vi "Save text file.vi"(8 "error in (no error)":errorcluster, 10 "Data":dbl, 11 "CSV Actor in":refnum<class "CSV Actor.lvclass">) -> (0 "error out":errorcluster, 3 "CSV Actor out":refnum<class "CSV Actor.lvclass">)   [LabVIEW 2020, in "CSV Actor.lvlib" / "CSV Actor.lvclass"]
uses:
  CSV Actor.lvclass
  <vilib>/Utility/file.llb/Write Delimited Spreadsheet (DBL).vi
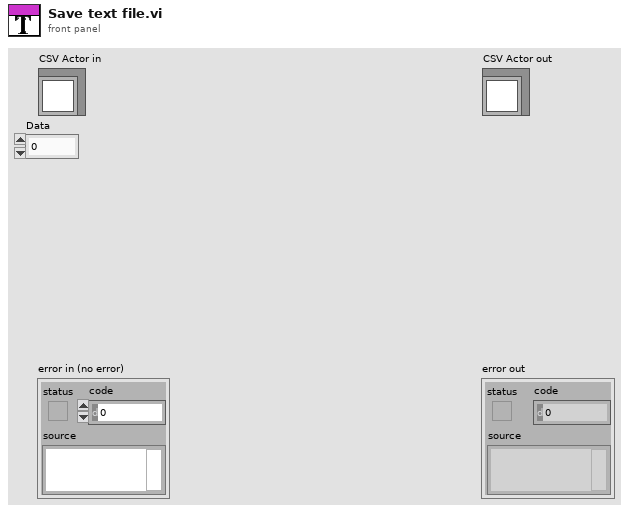
[diagram p1: front panel]
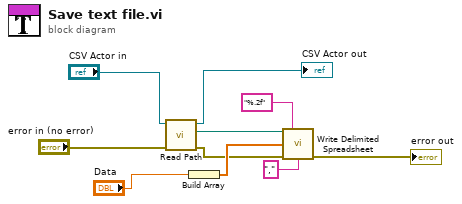
[diagram p0: block diagram]
diagram:
  n1 = call-dynamic "Read Path.vi"("error in (no error)"="error in (no error)", "Text Actor in"="CSV Actor in") -> ("error out"=w4:errorcluster, "Path"=w8:path, "Text Actor out"=→"CSV Actor out":refnum<class "CSV Actor.lvclass">)  [unwired: 7 in]
  n2 = Build Array("Data") -> (w6:dbl[])
  n3 = call-poly <vilib>:"Write Delimited Spreadsheet.vi"("file path (dialog if empty)"=w8, "format (%.3f)"="%.2f", "1D data"=w6, "error in (no error)"=w4, "delimiter (\\t)"="," ("delimiter (\\t)")) -> ("error out"=→"error out":errorcluster)  [unwired: 9 in, 1 out]
